vi "Define Channel Count.vi"(8 "error in":errorcluster, 11 "NI 9375 in":refnum<class "NI 9375.lvclass">) -> (0 "error out":errorcluster, 3 "NI 9375 out":refnum<class "NI 9375.lvclass">)   [LabVIEW 2017, in "Scan Engine Scripting.lvlib" / "NI 9375.lvclass"]
uses:
  NI 9375.lvclass
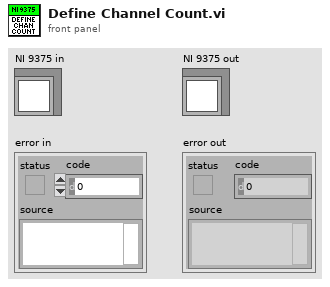
[diagram p1: front panel]
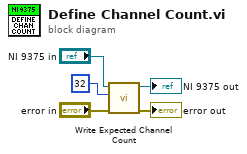
[diagram p0: block diagram]
diagram:
  n1 = call-dynamic "Write Expected Channel Count.vi"("error in"="error in", "expected channel count"=u8 32, "module in"="NI 9375 in") -> ("error out"=→"error out":errorcluster, "module out"=→"NI 9375 out":refnum<class "NI 9375.lvclass">)  [unwired: 7 in]
